vi "SetParam.vi"(8 "error in (no error)":errorcluster caption="entrée d'erreur (pas d'erreur)", 10 "MinMaxScaler":T1={"feature_range"={"min"=0.0, "max"=1.0}, "copy"=TRUE}, 11 "MinMaxScaler.lvclass":refnum<class "MinMaxScaler.lvclass">) -> (0 "error in (no error)":errorcluster caption="entrée d'erreur (pas d'erreur)", 3 "MinMaxScaler.lvclass":refnum<class "MinMaxScaler.lvclass">)   [LabVIEW 2020, in "MinMaxScaler.lvclass"]
doc: "Set Parameters"
uses:
  MinMaxScaler.lvclass
  MinMaxScaler.lvclass/MinMaxScaler.ctl
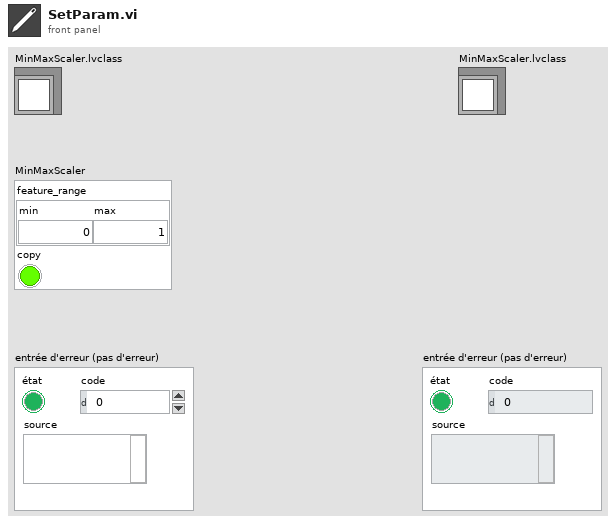
[diagram p1: front panel]
types:
  T1 = cluster{"feature_range":cluster{"min":dbl, "max":dbl}, "copy":bool}
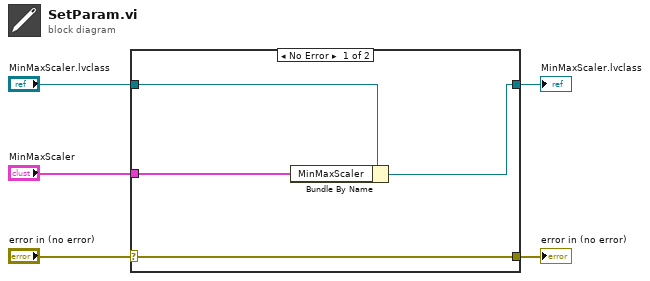
[diagram p0: block diagram]
diagram:
  n1 = case shown="No Error" "error in (no error)" {
    selector: "error in (no error)" -> [w9 w10]
    tunnel: [w9 w10] -> w4
    tunnel: [w7 w11] -> w2
    tunnel: "MinMaxScaler.lvclass" -> [w8 w11]
    tunnel: "MinMaxScaler" -> [w6 _]
    frame No Error {
      n2 = Bundle By Name(cluster=w8, "MinMaxScaler"=w6) -> (w7:refnum<class "MinMaxScaler.lvclass">)
    }
    frame Error {
    }
  }
  "error in (no error)" <- w4
  "MinMaxScaler.lvclass" <- w2
